vi "Data_Collection.vi"(11 "data":dynamicdata(waveform)) -> (1 "Scalar":dbl, 2 "Force":dynamicdata(graph), 3 "Dynamic Data":dynamicdata(waveform), 4 "Array":dbl[][](array[numeric]), 5 "Displacement":dynamicdata(graph))   [LabVIEW 2017]
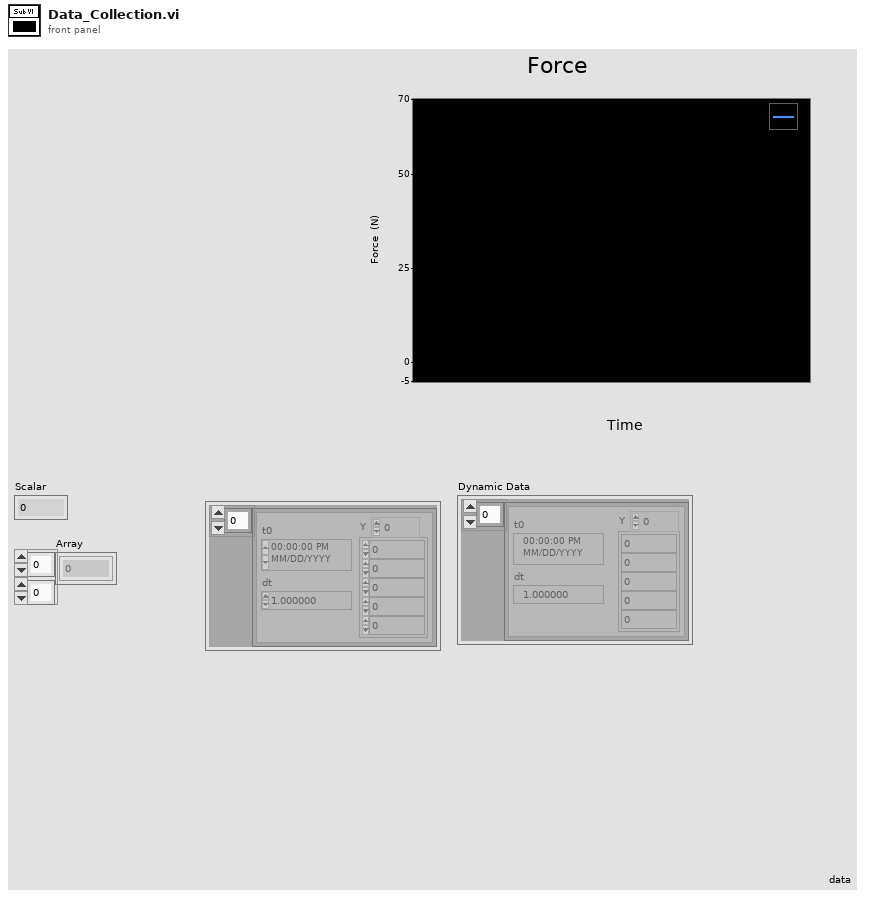
[diagram p1: front panel]
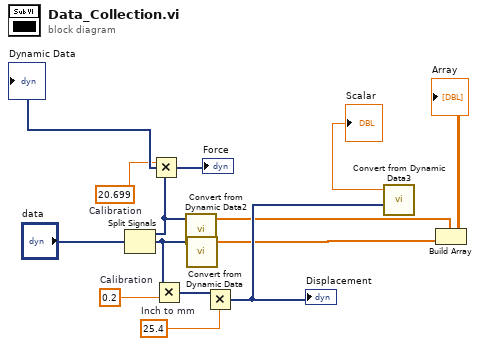
[diagram p0: block diagram]
diagram:
  w10 = 25.4  # Inch to mm
  w8 = 20.699  # Calibration
  w5 = 0.2  # Calibration
  n1 = Split Signals("data") -> (w7:dynamicdata, w6:dynamicdata)  [unwired: 3 in, 1 out]
  n2 = Multiply(x=w8, y=w7) -> (x*y=→"Force" →"Dynamic Data":dynamicdata)
  n3 = Multiply(x=w6, y=w5) -> (x*y=w9:dynamicdata)
  n4 = call "Convert from Dynamic Data2"("Dynamic Data Type"=w7) -> ("Array"=w2:dbl[])  [unwired: 3 in]
  n5 = call "Convert from Dynamic Data"("Dynamic Data Type"=w6) -> ("Array"=w3:dbl[])  [unwired: 3 in]
  n6 = Multiply(x=w9, y=w10) -> (x*y=w12:dynamicdata)
  "Displacement" <- w12
  n7 = call "Convert from Dynamic Data3"("Dynamic Data Type"=w12) -> ("Scalar"=→"Scalar":dbl)  [unwired: 3 in]
  n8 = Build Array(w2, w3) -> (→"Array":dbl[][])
